vi "Init.vi"(7 "family":string, 8 "error in":errorcluster, 9 "style":i32(ring)=1 items=["Regular"=0, "Bold"=1, "Italic"=2, "Underline"=4, "Strikeout"=8], 10 "emSize":sgl) -> (0 "error out":errorcluster, 3 "Font out":refnum<class "Font.lvclass">)   [LabVIEW 2024, in "SourceGrid.lvlib" / "Font.lvclass"]
uses:
  Font.lvclass
  Font.lvclass/Font.ctl
  System.Drawing
panel:
  in  "Font in":refnum<class "Font.lvclass">
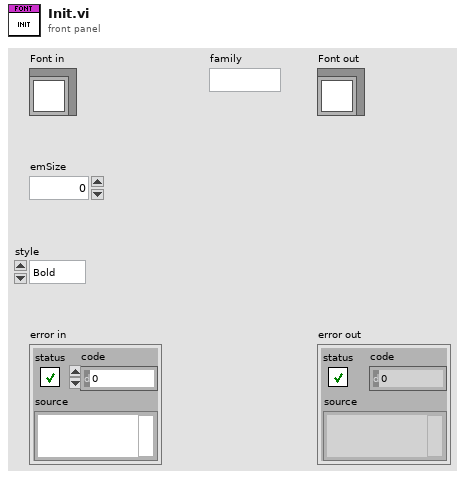
[diagram p1: front panel]
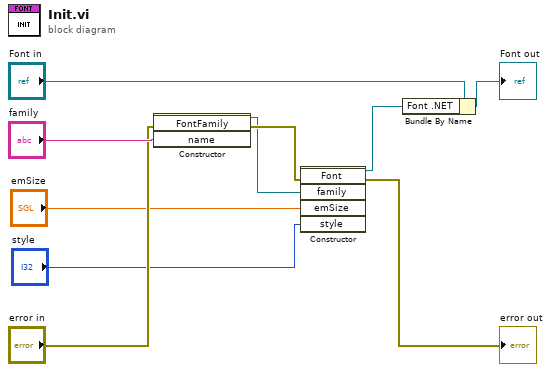
[diagram p0: block diagram]
diagram:
  n1 = constructor class="FontFamily" ("Constructor Font")(error in="error in", "name"="family") -> (reference out=w4:refnum<k24>, error out=w8:errorcluster)  [unwired: 2 in, 2 out]
  n2 = constructor class="Font" ("Constructor Font")(error in=w8, "family"=w4, "emSize"="emSize", "style"="style") -> (reference out=w1:refnum<k24>, error out=→"error out":errorcluster)  [unwired: 2 in, 4 out]
  n3 = Bundle By Name(cluster="Font in", "Font .NET"=w1) -> (→"Font out":refnum<class "Font.lvclass">)
